vi "Convert File Name to Track Names.vi"(11 "File Name":string) -> (3 "Track Names":T1)   [LabVIEW 2015]
doc: "Converts the given file name to 4 track names to be saved on the myRIO file system."
uses:
  Controls/Track File Names.ctl
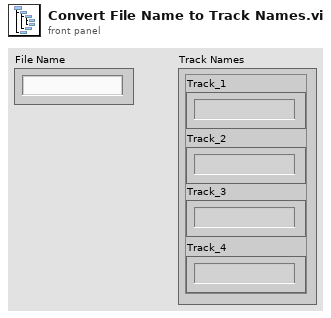
[diagram p1: front panel]
types:
  T1 = typedef "Track File Names.ctl" = cluster{"Track_1":string, "Track_2":string, "Track_3":string, "Track_4":string}
  T2 = cluster{"Track_1":string, "Track_2":string, "Track_3":string, "Track_4":string}
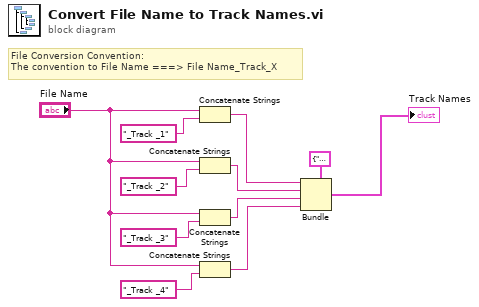
[diagram p0: block diagram]
diagram:
  # "File Conversion Convention:\nThe convention to File Name ===> File Name_Track_X"
  n1 = Concatenate Strings("File Name", "_Track _1" ("string")) -> (w5:string)
  n2 = Concatenate Strings("File Name", "_Track _2" ("string")) -> (w4:string)
  n3 = Concatenate Strings("File Name", "_Track _3" ("string")) -> (w3:string)
  n4 = Concatenate Strings("File Name", "_Track _4" ("string")) -> (w2:string)
  n5 = Bundle(cluster=T2 {"Track_1"="", "Track_2"="", "Track_3"="", "Track_4"=""}, "Track_1"=w5, "Track_2"=w4, "Track_3"=w3, "Track_4"=w2) -> (→"Track Names":T2)
